vi "Termo_1.5__.vi"() -> ()   [LabVIEW 2013]
doc: "Программа мониторинга температуры"
uses:
  <vilib>/Utility/error.llb/DialogType.ctl
panel:
  out "Связь с прибором":bool
  out "Configuring ADC?":bool
  in  "Tab Control":enum32{"Измерения", "Настройки", "Kоэффициенты"}(tab)
  in  "Autoscale":bool=TRUE
  out "часы":string="0"
  in  "Т max":u16=300 min=2 max=500 step=1
  in  "Т min":u16=3 min=1 max=350
  out "T2":dbl format="%.2f"
  out "T4":dbl format="%.2f"
  out "T1":dbl format="%.2f"
  out "T3":dbl format="%.2f"
  out "T6":dbl format="%.2f"
  out "T8":dbl format="%.2f"
  out "T5":dbl format="%.2f"
  out "T7":dbl format="%.2f"
  out "disconnected":bool
  in  "Добавить время":dbl(ring)=300.0 items=["1 мин."=60.0, "5 мин."=300.0, "20 мин."=1200.0]
  in  "Стоп измер.":bool
  in  "Старт измер.":bool
  in  "stop":bool
  out "R2":dbl format="%.2f"
  out "R4":dbl format="%.2f"
  out "R1":dbl format="%.2f"
  out "R3":dbl format="%.2f"
  out "мин.":string="1"
  in  "xScale +":bool
  in  "xScale -":bool
  in  "R max":u16=6000 min=2 max=10000 step=1
  in  "R min":u16=100 min=1 max=350
  in  "GraphLookB":bool
  out "R6":dbl format="%.2f"
  out "R8":dbl format="%.2f"
  out "R5":dbl format="%.2f"
  out "R7":dbl format="%.2f"
  in  "1_ch_visible":bool=TRUE
  in  "2_ch_visible":bool=TRUE
  in  "3_ch_visible":bool=TRUE
  in  "4_ch_visible":bool=TRUE
  in  "5_ch_visible":bool=TRUE
  in  "6_ch_visible":bool=TRUE
  in  "7_ch_visible":bool=TRUE
  in  "8_ch_visible":bool=TRUE
  in  "ADC_dyn_range":T1(ring)=enum."± 0.625 В"
  out "История операций":string
  in  "Buf_size":u8=16 min=1 max=128
  in  "SPS":T2(ring)
  in  "disconnect":bool
  in  "connect":bool
  in  "IP-адрес":string="192.168.127.254"
  in  "порт":u16=4001
  out "Расположение\n файла":path caption="Расположение файла"
  in  "load_coeff.":bool caption="Disconn"
  in  "save_coeff.":bool caption="Disconn"
  in  "Coeff_cl_ch8":T3 caption="Канал 8" {"R" format="%#_16g"; "k7" format="%#_16g"; "k6" format="%#_16g"; "k5" format="%#_16g"; "k4" format="%#_16g"; "k3" format="%#_16g"; "k2" format="%#_16g"; "k1" format="%#_16g"}
  in  "Coeff_cl_ch7":T3 caption="Канал 7" {"R" format="%#_16g"; "k7" format="%#_16g"; "k6" format="%#_16g"; "k5" format="%#_16g"; "k4" format="%#_16g"; "k3" format="%#_16g"; "k2" format="%#_16g"; "k1" format="%#_16g"}
  in  "Coeff_cl_ch6":T3 caption="Канал 6" {"R" format="%#_16g"; "k7" format="%#_16g"; "k6" format="%#_16g"; "k5" format="%#_16g"; "k4" format="%#_16g"; "k3" format="%#_16g"; "k2" format="%#_16g"; "k1" format="%#_16g"}
  in  "Coeff_cl_ch5":T3 caption="Канал 5" {"R" format="%#_16g"; "k7" format="%#_16g"; "k6" format="%#_16g"; "k5" format="%#_16g"; "k4" format="%#_16g"; "k3" format="%#_16g"; "k2" format="%#_16g"; "k1" format="%#_16g"}
  in  "Coeff_cl_ch4":T3 caption="Канал 4" {"R" format="%#_16g"; "k7" format="%#_16g"; "k6" format="%#_16g"; "k5" format="%#_16g"; "k4" format="%#_16g"; "k3" format="%#_16g"; "k2" format="%#_16g"; "k1" format="%#_16g"}
  in  "Coeff_cl_ch3":T3 caption="Канал 3" {"R" format="%#_16g"; "k7" format="%#_16g"; "k6" format="%#_16g"; "k5" format="%#_16g"; "k4" format="%#_16g"; "k3" format="%#_16g"; "k2" format="%#_16g"; "k1" format="%#_16g"}
  in  "Coeff_cl_ch2":T3 caption="Канал 2" {"R" format="%#_16g"; "k7" format="%#_16g"; "k6" format="%#_16g"; "k5" format="%#_16g"; "k4" format="%#_16g"; "k3" format="%#_16g"; "k2" format="%#_16g"; "k1" format="%#_16g"}
  in  "Coeff_cl_ch1":T3 caption="Канал 1" {"R" format="%#_16g"; "k7" format="%#_16g"; "k6" format="%#_16g"; "k5" format="%#_16g"; "k4" format="%#_16g"; "k3" format="%#_16g"; "k2" format="%#_16g"; "k1" format="%#_16g"}
  out "Сутки":string
  out "счетчик":u32=4001
  in  "Запись в файл":bool
  out "сек.":string="0"
  out "Graphs T":dynamicdata(graph) caption="Температура, К"
  out "refnum out":refnum<file>
  in  "File header exist?":bool caption="Disconn"
  out "connection ID":refnum<k5>
  out "Graphs R":dynamicdata(graph) caption="Сопротивление, Ом"
  out "Расположение файла":path
  # "T [K]"
  # "Канал"
  # "R [Ом]"
  # "1"
  # "2"
  # "3"
  # "4"
  # "5"
  # "6"
  # "7"
  # "8"
  # "Измерения"
  # "Шкала Т"
  # "Шкала R"
  # "Интервал просмотра"
  # ":"
  # "Скорость измерений"
  # "SPS = Samples Per Second"
  # "Динамический диапазон"
  # "Размер буфера усреднения"
  # "Подключение"
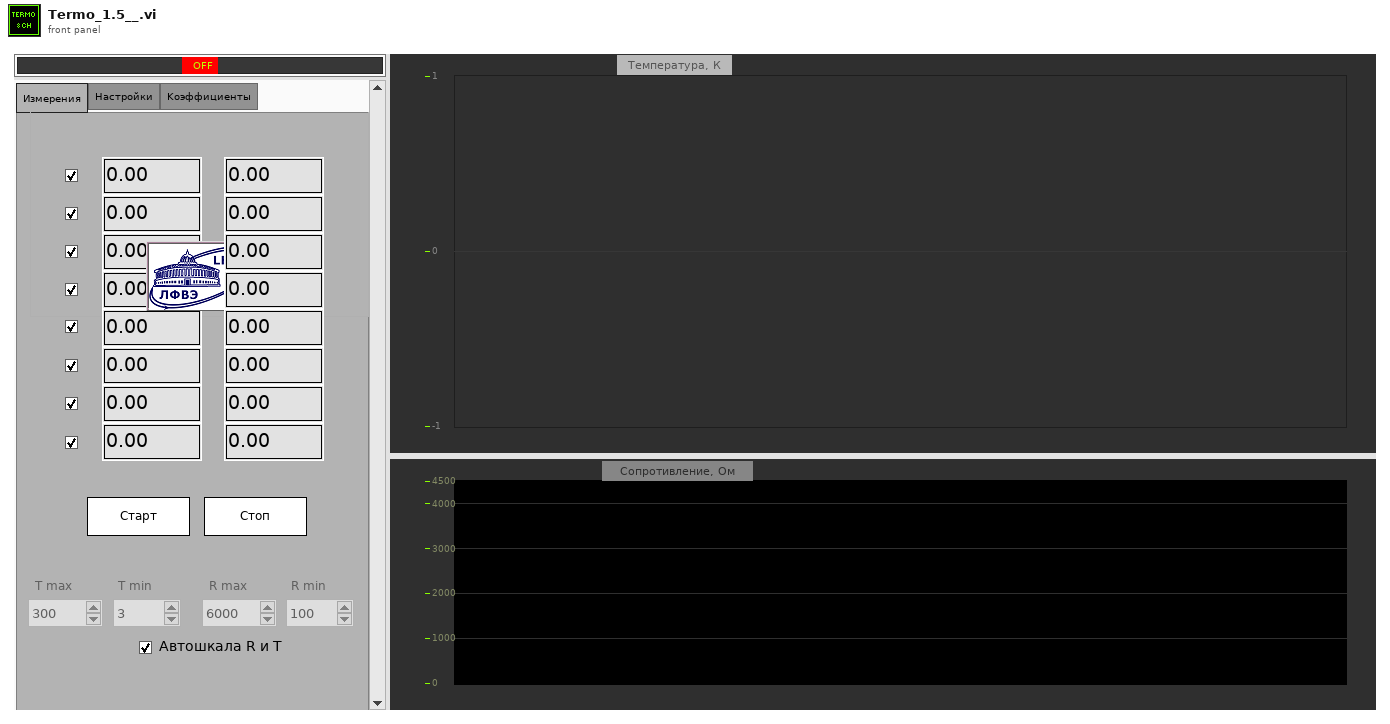
[diagram p1: front panel]
types:
  T1 = enum16{"± 5 В", "± 2.5 В", "± 1.25 В", "± 0.625 В", "± 312.5 мВ", "± 156.25 мВ", "± 78.125 мВ"}
  T2 = enum16{"2,5 SPS", "5 SPS", "10 SPS", "25 SPS", "50 SPS", "100 SPS", "500 SPS", "1 kSPS", "3,75 kSPS"}
  T3 = cluster{"k1":ext, "k2":ext, "k3":ext, "k4":ext, "k5":ext, "k6":ext, "k7":ext, "R":ext}
  T4 = enum32{"Page Enabled", "Page Disabled", "Page Disabled & Grayed"}
  T5 = enum16{"Standard", "Buffered", "CRLF", "Immediate"}
  T6 = typedef "DialogType.ctl" = u16
  T7 = typedef "LVDateTimeRec.ctl" = cluster{"fractional second":dbl, "second":i32, "minute":i32, "hour":i32, "day of month":i32, "month":i32, "year":i32, "day of week":i32, "day of year":i32, "DST":i32}
  T8 = cluster{" R1":dbl, " R2":dbl, " R3":dbl, " R4":dbl, " R5":dbl, "R6":dbl, " R7":dbl, "R8":dbl}
  T9 = cluster{" T1":dbl, "T2":dbl, "T3":dbl, "T4":dbl, " T5":dbl, "T6":dbl, "T7":dbl, "T8":dbl}
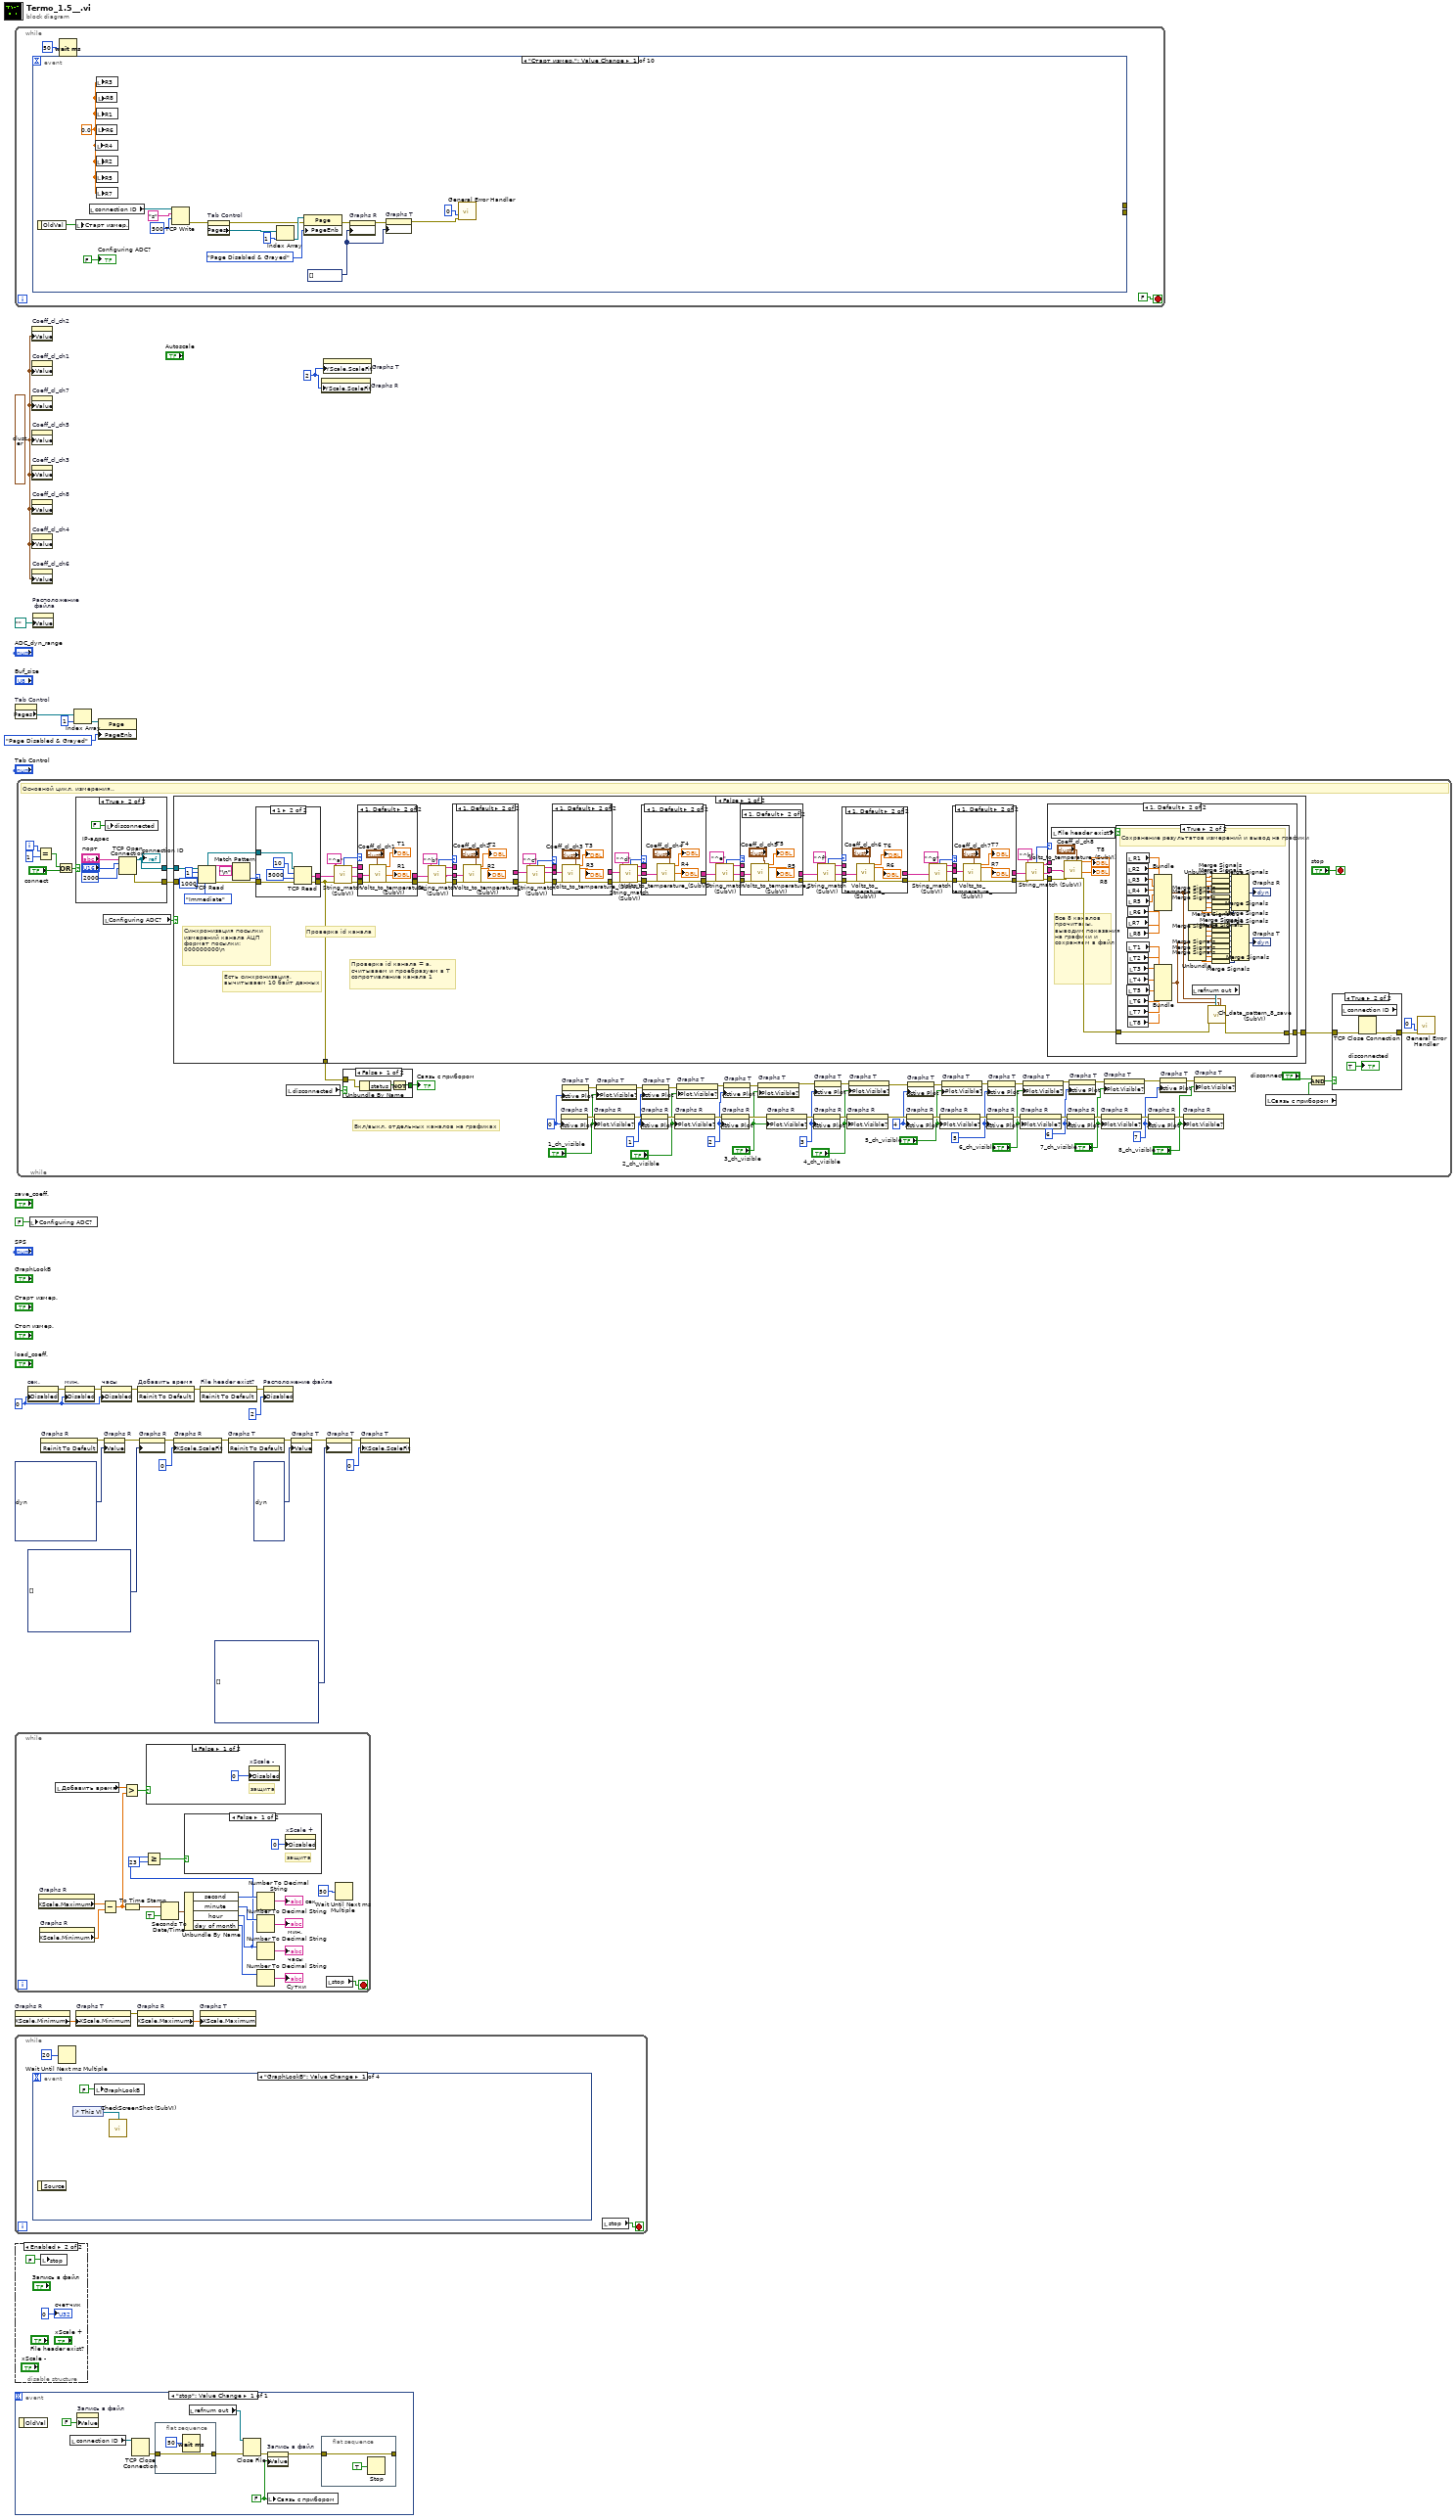
[diagram p0: block diagram]
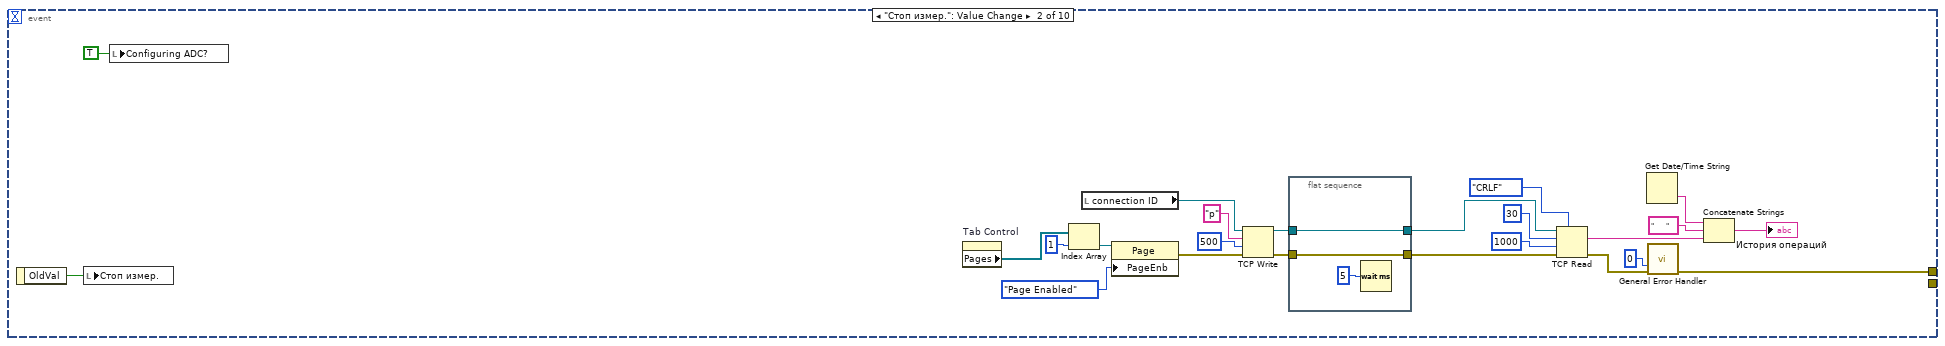
[diagram p2: hidden frame]
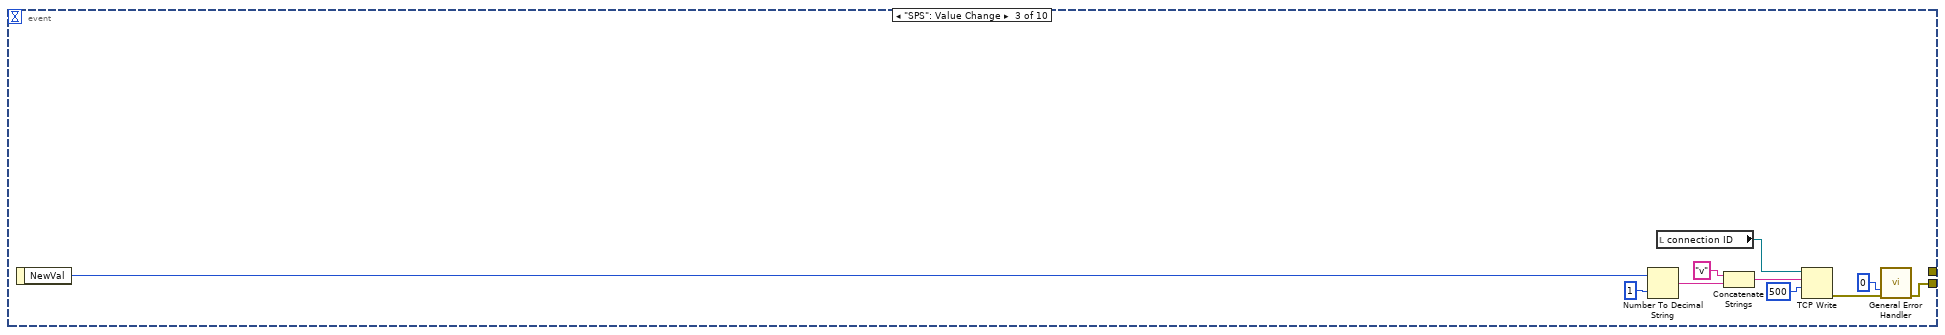
[diagram p3: hidden frame]
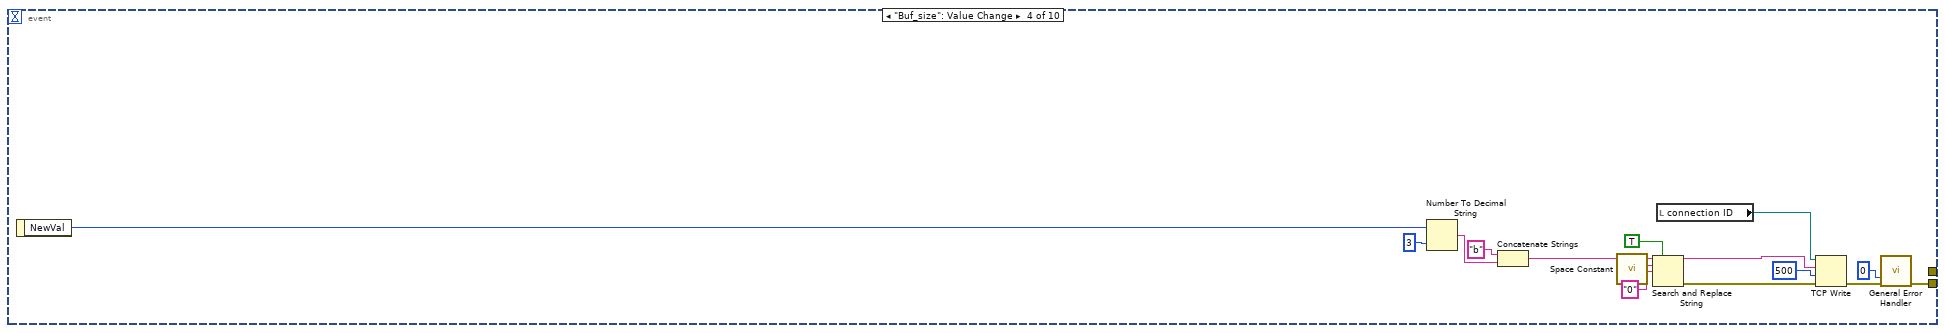
[diagram p4: hidden frame]
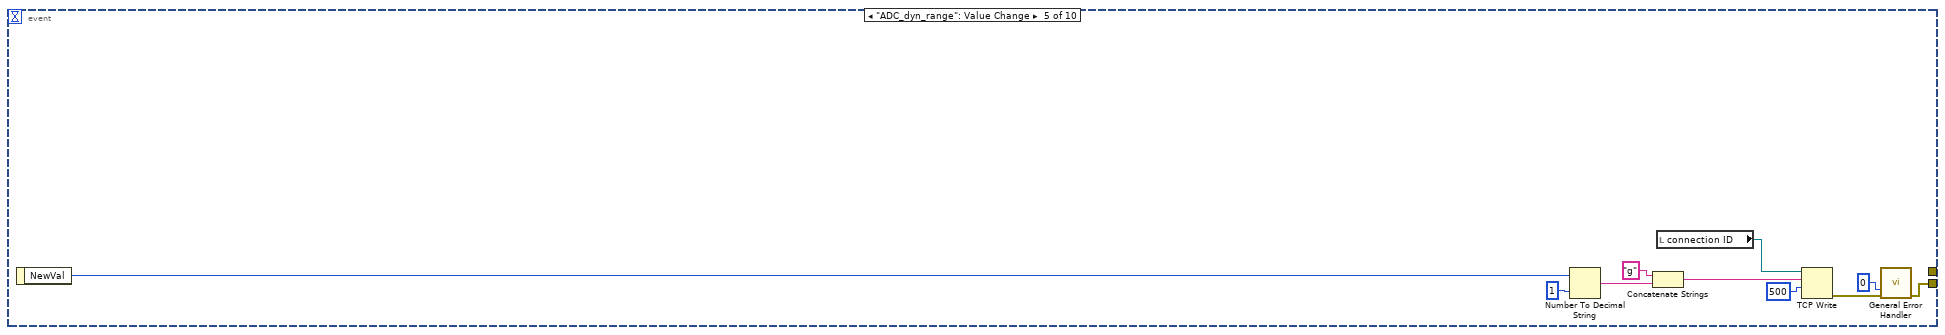
[diagram p5: hidden frame]
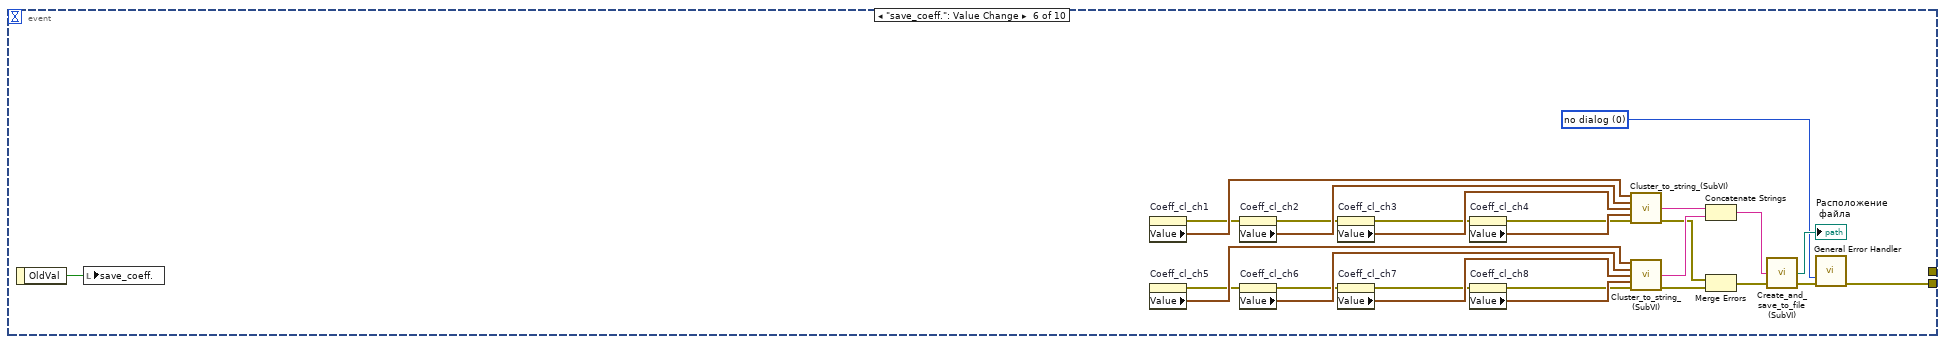
[diagram p6: hidden frame]
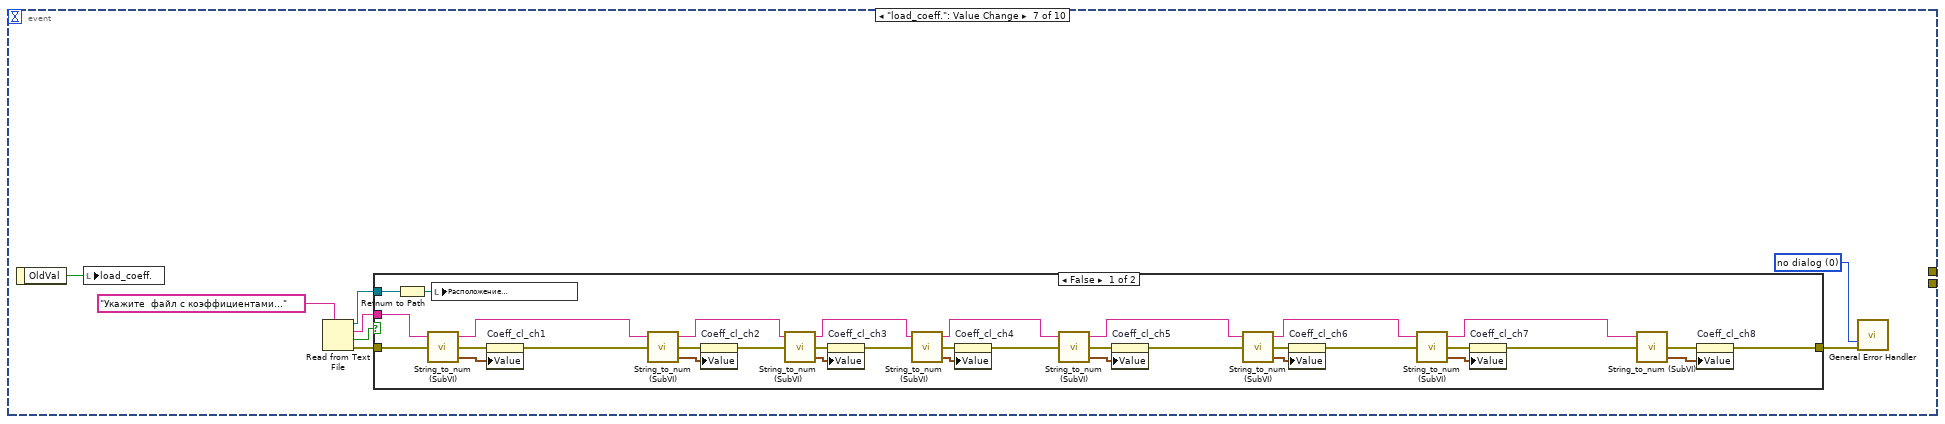
[diagram p7: hidden frame]
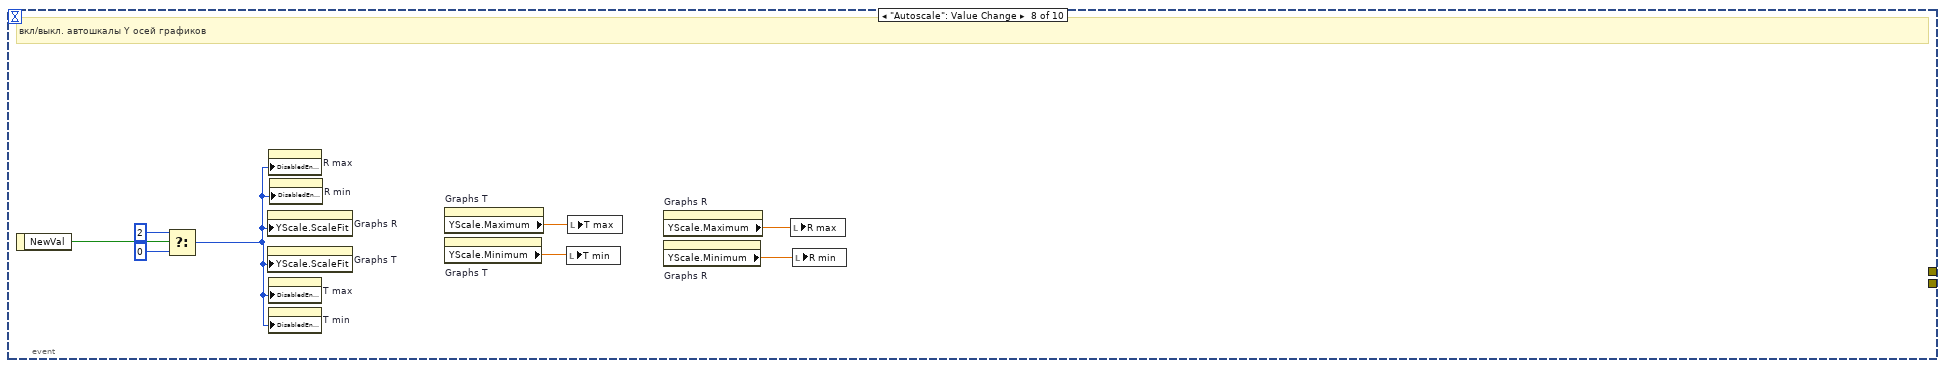
[diagram p9: hidden frame]
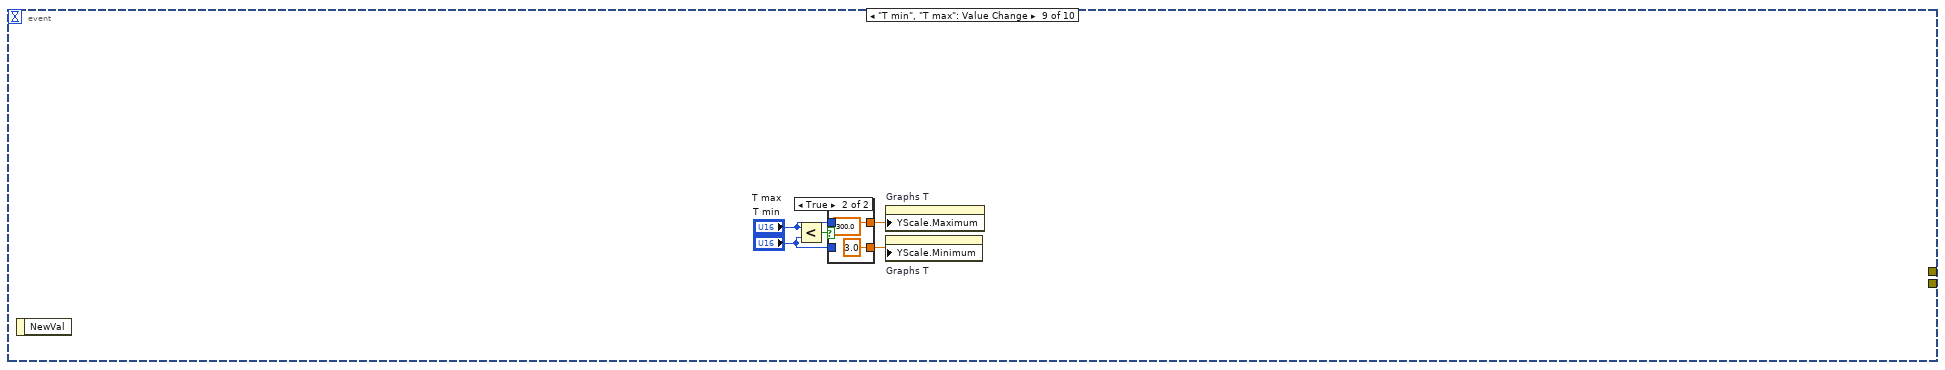
[diagram p10: hidden frame]
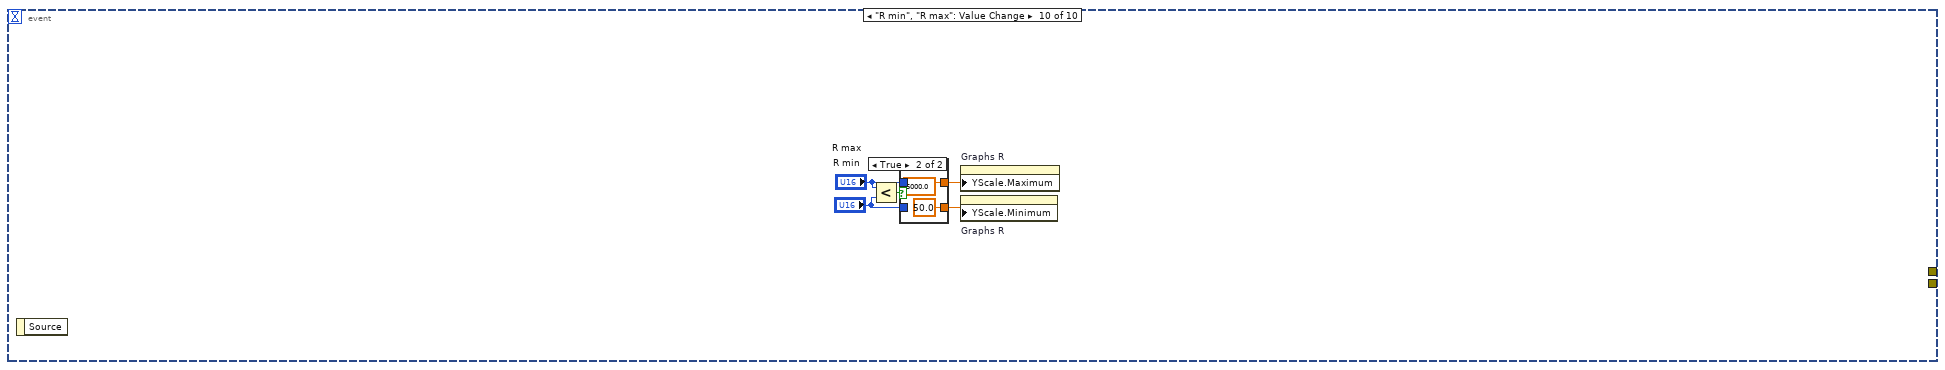
[diagram p12: hidden frame]
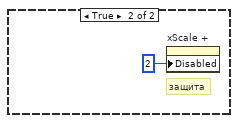
[diagram p14: hidden frame]
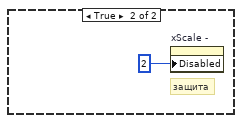
[diagram p15: hidden frame]
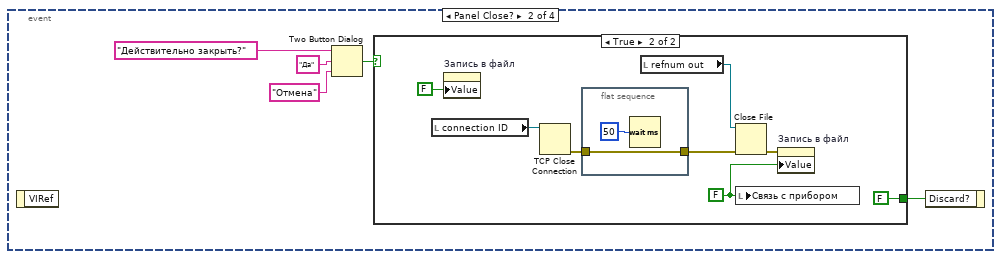
[diagram p17: hidden frame]
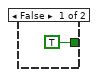
[diagram p18: hidden frame]
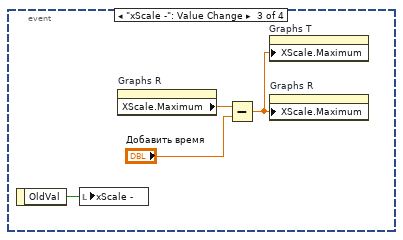
[diagram p19: hidden frame]
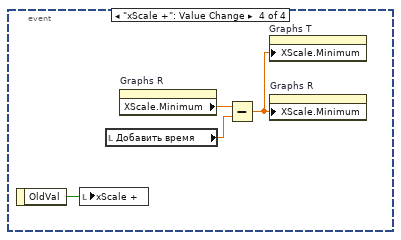
[diagram p20: hidden frame]
diagram:
  w1 = u8 2 ("Y Scale.Scale Fit")
  w3 = T3 {"k1"=0.0, "k2"=0.0, "k3"=0.0, "k4"=0.0, "k5"=0.0, "k6"=0.0, "k7"=0.0, "R"=0.0} ("Coeff_cl_ch2")
  w30 = u8 0 ("Disabled")
  n1 = while {
    stop <- FALSE stop-if-true
    n2 = event shown="[0] \"Старт измер.\": Value Change" {
      selector: _ -> [_ _ _ _ _ _ _ _ _ _]
      dyn-events: _ -> [_ _ _ _ _ _ _ _ _ _]
      timeout: _ -> [_ _ _ _ _ _ _ _ _ _]
      tunnel: [_ w53 _ _ _ _ _ _ _ _] -> _
      tunnel: [_ _ w79 w89 w103 w114 _ _ _ _] -> _
      event "Старт измер.": Value Change {
        w41 = 0.0 ("3")
        w35 = dynamicdata[] [] ("History Data")
        n3 = event-data() -> ("OldVal"=w50:bool)  [unwired: 1 in]
        n4 = local write "Старт измер."(w50) -> ()
        n5 = local read "connection ID"() -> (w46:refnum<k5>)
        n6 = local write "R4"(w41) -> ()
        n7 = local write "R3"(w41) -> ()
        n8 = local write "R1"(w41) -> ()
        n9 = local write "R2"(w41) -> ()
        n10 = local write "R5"(w41) -> ()
        n11 = local write "R7"(w41) -> ()
        n12 = local write "R8"(w41) -> ()
        n13 = local write "R6"(w41) -> ()
        n14 = TCP Write(connection ID=w46, data in="s", 9:500 ("timeout ms (25000)")) -> (error out=w39:errorcluster)  [unwired: 1 in, 2 out]
        n15 = property on="Tab Control" class="TabCtl (strict)"(error in=w39) -> (error out=w38:errorcluster, "Pages"=w45:refnum<vi>[])  [unwired: 1 in, 1 out]
        n16 = Index Array(array=w45, index=1) -> (element=w44:refnum<vi>)
        n17 = property class="Page"(reference=w44, error in=w38, "PageEnb"=T4."Page Disabled & Grayed" ("Page Enabled State")) -> (error out=w40:errorcluster)  [unwired: 1 out]
        n18 = property on="Graphs R" class="WFChart (strict)"(error in=w40, "History Data"=w35) -> (error out=w36:errorcluster)  [unwired: 1 in, 1 out]
        n19 = property on="Graphs T" class="WFChart (strict)"(error in=w36, "History Data"=w35) -> (error out=w34:errorcluster)  [unwired: 1 in, 1 out]
        n20 = call <vilib>:"General Error Handler.vi"("type of dialog (OK msg:1)"=0 ("timeout ms (25000)"), "error in (no error)"=w34) -> ()  [unwired: 9 in, 5 out]
        "Configuring ADC?" <- FALSE ("TCP_Wr_fl")
      }
      event "Стоп измер.": Value Change {
        n21 = event-data() -> ("OldVal"=w74:bool)  [unwired: 1 in]
        n22 = local write "Стоп измер."(w74) -> ()
        n23 = local write "Configuring ADC?"(TRUE ("TCP_Wr_fl")) -> ()
        n24 = property on="Tab Control" class="TabCtl (strict)"() -> ("Pages"=w69:refnum<vi>[])  [unwired: 2 in, 2 out]
        n25 = Index Array(array=w69, index=1) -> (element=w68:refnum<vi>)
        n26 = local read "connection ID"() -> (w71:refnum<k5>)
        n27 = property class="Page"(reference=w68, "PageEnb"=T4."Page Enabled" ("Page Enabled State")) -> (error out=w51:errorcluster)  [unwired: 1 in, 1 out]
        n28 = TCP Write(connection ID=w71, data in="p", error in (no error)=w51, 9:500 ("timeout ms (25000)")) -> (connection ID out=w61:refnum<k5>, error out=w59:errorcluster)  [unwired: 1 out]
        n29 = flat-sequence {
          tunnel: [w76] -> w62
          tunnel: w61 -> [w76]
          tunnel: [w75] -> w60
          tunnel: w59 -> [w75]
          frame #0 {
            n30 = Wait (ms)(milliseconds to wait=u32 5) -> ()  [unwired: 1 out]
          }
        }
        n31 = TCP Read(connection ID=w62, bytes to read=30, error in (no error)=w60, 7:T5."CRLF" ("mode (standard)"), 9:1000 ("timeout ms (25000)")) -> (data out=w56:string, error out=w54:errorcluster)  [unwired: 1 out]
        n32 = Get Date/Time String() -> (time string=w58:string)  [unwired: 3 in, 1 out]
        n33 = call <vilib>:"General Error Handler.vi"("type of dialog (OK msg:1)"=0 ("timeout ms (25000)"), "error in (no error)"=w54) -> ("error out"=w53:errorcluster)  [unwired: 9 in, 4 out]
        n34 = Concatenate Strings(w58, "      " ("string"), w56) -> (→"История операций":string)
      }
      event "SPS": Value Change {
        n35 = event-data() -> ("NewVal"=w84:T2)  [unwired: 1 in]
        n36 = Number To Decimal String(number=w84, width (-)=i16 1) -> (decimal integer string=w82:string)
        n37 = local read "connection ID"() -> (w86:refnum<k5>)
        n38 = Concatenate Strings("v" ("data in"), w82) -> (w81:string)
        n39 = TCP Write(connection ID=w86, data in=w81, 9:500 ("timeout ms (25000)")) -> (error out=w80:errorcluster)  [unwired: 1 in, 2 out]
        n40 = call <vilib>:"General Error Handler.vi"("type of dialog (OK msg:1)"=0 ("timeout ms (25000)"), "error in (no error)"=w80) -> ("error out"=w79:errorcluster)  [unwired: 9 in, 4 out]
      }
      event "Buf_size": Value Change {
        n41 = event-data() -> ("NewVal"=w99:u8)  [unwired: 1 in]
        n42 = Number To Decimal String(number=w99, width (-)=i16 3) -> (decimal integer string=w97:string)
        n43 = Concatenate Strings("b" ("data in"), w97) -> (w96:string)
        n44 = call <vilib>:"Space Constant.vi"() -> ("String"=w94:string)
        n45 = Search and Replace String(replace all?=TRUE ("replace all? (F)"), input string=w96, search string=w94, replace string="0" ("replace string (\"\")")) -> (result string=w95:string, error out=w91:errorcluster)  [unwired: 4 in, 2 out]
        n46 = local read "connection ID"() -> (w101:refnum<k5>)
        n47 = TCP Write(connection ID=w101, data in=w95, error in (no error)=w91, 9:500 ("timeout ms (25000)")) -> (error out=w90:errorcluster)  [unwired: 2 out]
        n48 = call <vilib>:"General Error Handler.vi"("type of dialog (OK msg:1)"=0 ("timeout ms (25000)"), "error in (no error)"=w90) -> ("error out"=w89:errorcluster)  [unwired: 9 in, 4 out]
      }
      event "ADC_dyn_range": Value Change {
        n49 = event-data() -> ("NewVal"=w109:T1)  [unwired: 1 in]
        n50 = Number To Decimal String(number=w109, width (-)=i16 1) -> (decimal integer string=w107:string)
        n51 = Concatenate Strings("g" ("data in"), w107) -> (w106:string)
        n52 = local read "connection ID"() -> (w111:refnum<k5>)
        n53 = TCP Write(connection ID=w111, data in=w106, 9:500 ("timeout ms (25000)")) -> (error out=w104:errorcluster)  [unwired: 1 in, 2 out]
        n54 = call <vilib>:"General Error Handler.vi"("type of dialog (OK msg:1)"=0 ("timeout ms (25000)"), "error in (no error)"=w104) -> ("error out"=w103:errorcluster)  [unwired: 9 in, 4 out]
      }
      event "save_coeff.": Value Change {
        w113 = T6 0 items=["no dialog", "OK message", "continue or stop message", "OK message + warnings", "continue/stop + warnings"] ("type of dialog (OK msg:1)")
        n55 = event-data() -> ("OldVal"=w120:bool)  [unwired: 1 in]
        n56 = local write "save_coeff."(w120) -> ()
        n57 = property on="Coeff_cl_ch1" class="Clust (strict)"() -> (error out=w127:errorcluster, "Value"=w135:T3)  [unwired: 2 in, 1 out]
        n58 = property on="Coeff_cl_ch5" class="Clust (strict)"() -> (error out=w124:errorcluster, "Value"=w131:T3)  [unwired: 2 in, 1 out]
        n59 = property on="Coeff_cl_ch2" class="Clust (strict)"(error in=w127) -> (error out=w126:errorcluster, "Value"=w134:T3)  [unwired: 1 in, 1 out]
        n60 = property on="Coeff_cl_ch6" class="Clust (strict)"(error in=w124) -> (error out=w123:errorcluster, "Value"=w130:T3)  [unwired: 1 in, 1 out]
        n61 = property on="Coeff_cl_ch3" class="Clust (strict)"(error in=w126) -> (error out=w125:errorcluster, "Value"=w133:T3)  [unwired: 1 in, 1 out]
        n62 = property on="Coeff_cl_ch7" class="Clust (strict)"(error in=w123) -> (error out=w122:errorcluster, "Value"=w129:T3)  [unwired: 1 in, 1 out]
        n63 = property on="Coeff_cl_ch4" class="Clust (strict)"(error in=w125) -> (error out=w117:errorcluster, "Value"=w132:T3)  [unwired: 1 in, 1 out]
        n64 = property on="Coeff_cl_ch8" class="Clust (strict)"(error in=w122) -> (error out=w116:errorcluster, "Value"=w128:T3)  [unwired: 1 in, 1 out]
        n65 = call "Cluster_to_string_(SubVI).vi"("input cluster 1"=w135, "input cluster 2"=w134, "input cluster 3"=w133, "input cluster 4"=w132, "error in"=w117) -> ("string of coefficients"=w138:string, "error out"=w119:errorcluster)  [unwired: 9 in]
        n66 = call "Cluster_to_string_(SubVI).vi"("input cluster 1"=w131, "input cluster 2"=w130, "input cluster 3"=w129, "input cluster 4"=w128, "error in"=w116) -> ("string of coefficients"=w139:string, "error out"=w118:errorcluster)  [unwired: 9 in]
        n67 = Concatenate Strings(w138, w139) -> (w121:string)
        n68 = Merge Errors(w119, w118) -> (w137:errorcluster)
        n69 = call "Create_and_save_to_file (SubVI).vi"("input string"=w121, "error in"=w137) -> ("Текущее расположение файла"=→"Расположение\n файла":path, "error out"=w115:errorcluster)  [unwired: 4 in]
        n70 = call <vilib>:"General Error Handler.vi"("type of dialog (OK msg:1)"=w113, "error in (no error)"=w115) -> ("error out"=w114:errorcluster)  [unwired: 9 in, 4 out]
      }
      event "load_coeff.": Value Change {
        w141 = T6 0 items=["no dialog", "OK message", "continue or stop message", "OK message + warnings", "continue/stop + warnings"] ("type of dialog (OK msg:1)")
        n71 = event-data() -> ("OldVal"=w147:bool)  [unwired: 1 in]
        n72 = local write "load_coeff."(w147) -> ()
        n73 = Read from Text File(prompt (Open existing file)="Укажите  файл с коэффициентами...") -> (refnum out=w140:refnum<file>, text=w144:string, cancelled=w143:bool, error out=w145:errorcluster)  [unwired: 3 in]
        n74 = case shown="False" w143 {
          tunnel: w145 -> [w182 w183]
          tunnel: w144 -> [w181 _]
          tunnel: [w150 w183] -> w142
          tunnel: w140 -> [w149 _]
          frame False {
            n75 = Refnum to Path(1:w149) -> (0:w148:path)
            n76 = call "String_to_num (SubVI).vi"("String in"=w181, "error in"=w182) -> ("Rest of string OUT"=w177:string, "error out"=w179:errorcluster, "output cluster \nof coefficients"=w180:T3)  [unwired: 5 in]
            n77 = local write "Расположение\n файла"(w148) -> ()
            n78 = property on="Coeff_cl_ch1" class="Clust (strict)"(error in=w179, "Value"=w180) -> (error out=w178:errorcluster)  [unwired: 1 in, 1 out]
            n79 = call "String_to_num (SubVI).vi"("String in"=w177, "error in"=w178) -> ("Rest of string OUT"=w173:string, "error out"=w176:errorcluster, "output cluster \nof coefficients"=w175:T3)  [unwired: 5 in]
            n80 = property on="Coeff_cl_ch2" class="Clust (strict)"(error in=w176, "Value"=w175) -> (error out=w174:errorcluster)  [unwired: 1 in, 1 out]
            n81 = call "String_to_num (SubVI).vi"("String in"=w173, "error in"=w174) -> ("Rest of string OUT"=w170:string, "error out"=w172:errorcluster, "output cluster \nof coefficients"=w171:T3)  [unwired: 5 in]
            n82 = property on="Coeff_cl_ch3" class="Clust (strict)"(error in=w172, "Value"=w171) -> (error out=w169:errorcluster)  [unwired: 1 in, 1 out]
            n83 = call "String_to_num (SubVI).vi"("String in"=w170, "error in"=w169) -> ("Rest of string OUT"=w165:string, "error out"=w168:errorcluster, "output cluster \nof coefficients"=w167:T3)  [unwired: 5 in]
            n84 = property on="Coeff_cl_ch4" class="Clust (strict)"(error in=w168, "Value"=w167) -> (error out=w166:errorcluster)  [unwired: 1 in, 1 out]
            n85 = call "String_to_num (SubVI).vi"("String in"=w165, "error in"=w166) -> ("Rest of string OUT"=w161:string, "error out"=w163:errorcluster, "output cluster \nof coefficients"=w164:T3)  [unwired: 5 in]
            n86 = property on="Coeff_cl_ch5" class="Clust (strict)"(error in=w163, "Value"=w164) -> (error out=w162:errorcluster)  [unwired: 1 in, 1 out]
            n87 = call "String_to_num (SubVI).vi"("String in"=w161, "error in"=w162) -> ("Rest of string OUT"=w157:string, "error out"=w159:errorcluster, "output cluster \nof coefficients"=w160:T3)  [unwired: 5 in]
            n88 = property on="Coeff_cl_ch6" class="Clust (strict)"(error in=w159, "Value"=w160) -> (error out=w158:errorcluster)  [unwired: 1 in, 1 out]
            n89 = call "String_to_num (SubVI).vi"("String in"=w157, "error in"=w158) -> ("Rest of string OUT"=w154:string, "error out"=w155:errorcluster, "output cluster \nof coefficients"=w156:T3)  [unwired: 5 in]
            n90 = property on="Coeff_cl_ch7" class="Clust (strict)"(error in=w155, "Value"=w156) -> (error out=w153:errorcluster)  [unwired: 1 in, 1 out]
            n91 = call "String_to_num (SubVI).vi"("String in"=w154, "error in"=w153) -> ("error out"=w151:errorcluster, "output cluster \nof coefficients"=w152:T3)  [unwired: 5 in, 1 out]
            n92 = property on="Coeff_cl_ch8" class="Clust (strict)"(error in=w151, "Value"=w152) -> (error out=w150:errorcluster)  [unwired: 1 in, 1 out]
          }
          frame True {
          }
        }
        n93 = call <vilib>:"General Error Handler.vi"("type of dialog (OK msg:1)"=w141, "error in (no error)"=w142) -> ()  [unwired: 9 in, 5 out]
      }
      event "Autoscale": Value Change {
        # "вкл/выкл. автошкалы Y осей графиков"
        n94 = event-data() -> ("NewVal"=w191:bool)  [unwired: 1 in]
        n95 = Select(t=u8 2 ("Y Scale.Scale Fit"), s=w191, f=u8 0 ("Y Scale.Scale Fit")) -> (s? t:f=w188:u8)
        n96 = property on="Graphs R" class="WFChart (strict)"("YScale.ScaleFit"=w188) -> ()  [unwired: 2 in, 2 out]
        n97 = property on="Graphs T" class="WFChart (strict)"("YScale.ScaleFit"=w188) -> ()  [unwired: 2 in, 2 out]
        n98 = property on="R max" class="DigNum (strict)"("DisabledEnum"=w188) -> ()  [unwired: 2 in, 2 out]
        n99 = property on="Т max" class="DigNum (strict)"("DisabledEnum"=w188) -> ()  [unwired: 2 in, 2 out]
        n100 = property on="Т min" class="DigNum (strict)"("DisabledEnum"=w188) -> ()  [unwired: 2 in, 2 out]
        n101 = property on="R min" class="DigNum (strict)"("DisabledEnum"=w188) -> ()  [unwired: 2 in, 2 out]
        n102 = property on="Graphs T" class="WFChart (strict)"() -> ("YScale.Maximum"=w184:dbl)  [unwired: 2 in, 2 out]
        n103 = property on="Graphs T" class="WFChart (strict)"() -> ("YScale.Minimum"=w185:dbl)  [unwired: 2 in, 2 out]
        n104 = local write "Т min"(w185) -> ()
        n105 = local write "Т max"(w184) -> ()
        n106 = property on="Graphs R" class="WFChart (strict)"() -> ("YScale.Maximum"=w186:dbl)  [unwired: 2 in, 2 out]
        n107 = property on="Graphs R" class="WFChart (strict)"() -> ("YScale.Minimum"=w187:dbl)  [unwired: 2 in, 2 out]
        n108 = local write "R max"(w186) -> ()
        n109 = local write "R min"(w187) -> ()
      }
      event "Т min", "Т max": Value Change {
        n110 = event-data() -> ()  [unwired: 1 in, 1 out]
        n111 = Less?(x="Т max", y="Т min") -> (x < y?=w196:bool)
        n112 = case shown="True" w196 {
          tunnel: [w197 300.0 ("x+1")] -> w194
          tunnel: [w198 3.0 ("x+1")] -> w195
          tunnel: "Т max" -> [w197 _]
          tunnel: "Т min" -> [w198 _]
          frame False {
          }
          frame True {
          }
        }
        n113 = property on="Graphs T" class="WFChart (strict)"("YScale.Maximum"=w194) -> ()  [unwired: 2 in, 2 out]
        n114 = property on="Graphs T" class="WFChart (strict)"("YScale.Minimum"=w195) -> ()  [unwired: 2 in, 2 out]
      }
      event "R min", "R max": Value Change {
        n115 = event-data() -> ()  [unwired: 1 in, 1 out]
        n116 = Less?(x="R max", y="R min") -> (x < y?=w203:bool)
        n117 = case shown="True" w203 {
          tunnel: [w206 5000.0 ("x+1")] -> w205
          tunnel: [w207 50.0 ("x+1")] -> w204
          tunnel: "R max" -> [w206 _]
          tunnel: "R min" -> [w207 _]
          frame False {
          }
          frame True {
          }
        }
        n118 = property on="Graphs R" class="WFChart (strict)"("YScale.Maximum"=w205) -> ()  [unwired: 2 in, 2 out]
        n119 = property on="Graphs R" class="WFChart (strict)"("YScale.Minimum"=w204) -> ()  [unwired: 2 in, 2 out]
      }
    }
    n120 = Wait (ms)(milliseconds to wait=u32 50) -> ()  [unwired: 1 out]
  }
  n121 = property on="Tab Control" class="TabCtl (strict)"() -> ("Pages"=w15:refnum<vi>[])  [unwired: 2 in, 2 out]
  n122 = while {
    stop <- w229 stop-if-true
    n123 = property on="Graphs R" class="WFChart (strict)"() -> ("XScale.Maximum"=w228:dbl)  [unwired: 2 in, 2 out]
    n124 = property on="Graphs R" class="WFChart (strict)"() -> ("XScale.Minimum"=w227:dbl)  [unwired: 2 in, 2 out]
    n125 = local read "Добавить время"() -> (w225:dbl)
    n126 = Subtract(x=w228, y=w227) -> (x-y=w214:dbl)
    n127 = Greater?(x=w225, y=w214) -> (0:w226:bool)
    n128 = To Time Stamp(1:w214) -> (0:w223:timestamp)
    n129 = case shown="False" w226 {
      frame False {
        # "защита"
        n130 = property on="xScale -" class="Bool (strict)"("Disabled"=u8 0) -> ()  [unwired: 2 in, 2 out]
      }
      frame True {
        # "защита"
        n131 = property on="xScale -" class="Bool (strict)"("Disabled"=u8 2) -> ()  [unwired: 2 in, 2 out]
      }
    }
    n132 = Seconds To Date/Time(time stamp (now)=w223, to UTC (F)=TRUE) -> (date time rec=w222:T7)
    n133 = Unbundle By Name(w222) -> ("second"=w221:i32, "minute"=w220:i32, "hour"=w211:i32, "day of month"=w219:i32)
    n134 = Greater Or Equal?(x=w211, y=23) -> (x >= y?=w212:bool)
    n135 = case shown="False" w212 {
      frame False {
        # "защита"
        n136 = property on="xScale +" class="Bool (strict)"("Disabled"=u8 0) -> ()  [unwired: 2 in, 2 out]
      }
      frame True {
        # "защита"
        n137 = property on="xScale +" class="Bool (strict)"("Disabled"=u8 2) -> ()  [unwired: 2 in, 2 out]
      }
    }
    n138 = Number To Decimal String(number=w221) -> (decimal integer string=→"сек.":string)  [unwired: 1 out]
    n139 = Number To Decimal String(number=w220) -> (decimal integer string=→"мин.":string)  [unwired: 1 out]
    n140 = Number To Decimal String(number=w211) -> (decimal integer string=→"часы":string)  [unwired: 1 out]
    n141 = Number To Decimal String(number=w219) -> (decimal integer string=→"Сутки":string)  [unwired: 1 out]
    n142 = local read "stop"() -> (w229:bool)
    n143 = Wait Until Next ms Multiple(millisecond multiple=u32 50) -> ()  [unwired: 1 out]
  }
  n144 = property on="Graphs R" class="WFChart (strict)"() -> ("XScale.Minimum"=w6:dbl)  [unwired: 2 in, 2 out]
  n145 = while {
    stop <- w234 stop-if-true
    n146 = event shown="[0] \"GraphLookB\": Value Change" {
      selector: _ -> [_ _ _ _]
      dyn-events: _ -> [_ _ _ _]
      timeout: _ -> [_ _ _ _]
      event "GraphLookB": Value Change {
        n147 = event-data() -> ()  [unwired: 2 out]
        n148 = control-ref of="This VI"() -> (w236:refnum<vi>)
        n149 = local write "GraphLookB"(FALSE ("Снимок")) -> ()
        n150 = call "CheckScreenShot (SubVI).vi"("VI reference"=w236) -> ()  [unwired: 15 in]
      }
      event Panel Close? {
        n151 = event-data() -> ()  [unwired: 2 out]
        n152 = Two Button Dialog(message="Действительно закрыть?", 1:"Отмена" ("T button name (\"OK\")"), 2:"Да" ("T button name (\"OK\")")) -> (T button?=w242:bool)
        n153 = case shown="True" w242 {
          tunnel: [TRUE ("Discard?") FALSE ("Discard?")] -> w238
          frame False {
          }
          frame True {
            w248 = FALSE ("Запись в файл")
            n154 = local read "connection ID"() -> (w245:refnum<k5>)
            n155 = property on="Запись в файл" class="Bool (strict)"("Value"=FALSE ("Запись в файл")) -> ()  [unwired: 2 in, 2 out]
            n156 = TCP Close Connection(connection ID=w245) -> (error out=w251:errorcluster)  [unwired: 1 in, 2 out]
            n157 = flat-sequence {
              tunnel: [w252] -> w250
              tunnel: w251 -> [w252]
              frame #0 {
                n158 = Wait (ms)(milliseconds to wait=u32 50) -> ()  [unwired: 1 out]
              }
            }
            n159 = local read "refnum out"() -> (w247:refnum<file>)
            n160 = Close File(refnum=w247, error in=w250) -> (error out=w246:errorcluster)  [unwired: 1 out]
            n161 = local write "Связь с прибором"(w248) -> ()
            n162 = property on="Запись в файл" class="Bool (strict)"(error in=w246, "Value"=w248) -> ()  [unwired: 1 in, 2 out]
          }
        }
        n163 = event-data("Discard?"=w238) -> ()  [unwired: 1 in, 1 out]
      }
      event "xScale -": Value Change {
        n164 = event-data() -> ("OldVal"=w256:bool)  [unwired: 1 out]
        n165 = local write "xScale -"(w256) -> ()
        n166 = property on="Graphs R" class="WFChart (strict)"() -> ("XScale.Maximum"=w257:dbl)  [unwired: 2 in, 2 out]
        n167 = Subtract(x=w257, y="Добавить время") -> (x-y=w254:dbl)
        n168 = property on="Graphs T" class="WFChart (strict)"("XScale.Maximum"=w254) -> ()  [unwired: 2 in, 2 out]
        n169 = property on="Graphs R" class="WFChart (strict)"("XScale.Maximum"=w254) -> ()  [unwired: 2 in, 2 out]
      }
      event "xScale +": Value Change {
        n170 = event-data() -> ("OldVal"=w260:bool)  [unwired: 1 out]
        n171 = local write "xScale +"(w260) -> ()
        n172 = local read "Добавить время"() -> (w259:dbl)
        n173 = property on="Graphs R" class="WFChart (strict)"() -> ("XScale.Minimum"=w261:dbl)  [unwired: 2 in, 2 out]
        n174 = Subtract(x=w261, y=w259) -> (x-y=w258:dbl)
        n175 = property on="Graphs T" class="WFChart (strict)"("XScale.Minimum"=w258) -> ()  [unwired: 2 in, 2 out]
        n176 = property on="Graphs R" class="WFChart (strict)"("XScale.Minimum"=w258) -> ()  [unwired: 2 in, 2 out]
      }
    }
    n177 = Wait Until Next ms Multiple(millisecond multiple=u32 20) -> ()  [unwired: 1 out]
    n178 = local read "stop"() -> (w234:bool)
  }
  n179 = disable-structure shown="Enabled" {
    frame Disabled {
    }
    frame Enabled {
      n180 = local write "stop"(FALSE ("Boolean")) -> ()
      "счетчик" <- u32 0 ("счетчик")
    }
  }
  n181 = event shown="[0] \"stop\": Value Change" {
    selector: _ -> [_]
    dyn-events: _ -> [_]
    timeout: _ -> [_]
    event "stop": Value Change {
      w268 = FALSE ("Запись в файл")
      n182 = event-data() -> ()  [unwired: 1 in, 1 out]
      n183 = local read "connection ID"() -> (w265:refnum<k5>)
      n184 = property on="Запись в файл" class="Bool (strict)"("Value"=FALSE ("Запись в файл")) -> ()  [unwired: 2 in, 2 out]
      n185 = TCP Close Connection(connection ID=w265) -> (error out=w271:errorcluster)  [unwired: 1 in, 2 out]
      n186 = flat-sequence {
        tunnel: [w274] -> w270
        tunnel: w271 -> [w274]
        frame #0 {
          n187 = Wait (ms)(milliseconds to wait=u32 50) -> ()  [unwired: 1 out]
        }
      }
      n188 = local read "refnum out"() -> (w267:refnum<file>)
      n189 = Close File(refnum=w267, error in=w270) -> (error out=w266:errorcluster)  [unwired: 1 out]
      n190 = property on="Запись в файл" class="Bool (strict)"(error in=w266, "Value"=w268) -> (error out=w264:errorcluster)  [unwired: 1 in, 1 out]
      n191 = local write "Связь с прибором"(w268) -> ()
      n192 = flat-sequence {
        tunnel: w264 -> [w273]
        tunnel: [w273] -> _
        frame #0 {
          n193 = Stop(stop? (T)=TRUE) -> ()
        }
      }
    }
  }
  n194 = while {
    i -> [w336]
    stop <- "stop" stop-if-true
    w279 = u32 7 ("Active Plot")
    w281 = u32 6 ("Active Plot")
    w283 = u32 5 ("Active Plot")
    w286 = u32 4 ("Active Plot")
    w296 = u32 3 ("Active Plot")
    w299 = u32 2 ("Active Plot")
    w302 = u32 1 ("Active Plot")
    w307 = u32 0 ("Active Plot")
    # "Вкл/выкл. отдельных каналов на графиках"
    # "Основной цикл, измерения.."
    n195 = Equal?(x=w336, y=1) -> (x = y?=w337:bool)
    n196 = Or(x=w337, y="connect") -> (x .or. y?=w319:bool)
    n197 = case shown="True" w319 {
      tunnel: [_ w351] -> w317
      tunnel: [w349 w352] -> w320
      frame False {
        n198 = local read "connection ID"() -> (w349:refnum<k5>)
      }
      frame True {
        n199 = local write "disconnected"(FALSE ("disconnected")) -> ()
        n200 = TCP Open Connection(address="IP-адрес", remote port or service name="порт", timeout ms (60000)=2000) -> (connection ID=w352:refnum<k5>, error out=w351:errorcluster)  [unwired: 1 in, 1 out]
        "connection ID" <- w352
      }
    }
    n201 = local read "Configuring ADC?"() -> (w311:bool)
    n202 = case shown="False" w311 {
      tunnel: [w356 w555] -> w277
      tunnel: w317 -> [w417 w555]
      tunnel: w320 -> [w416 _]
      tunnel: [w357 w555] -> w309
      frame False {
        # "Проверка id канала = a,\nсчитываем и проебразуем в Т\nсопротивление канала 1"
        # "Есть синхронизация, \nвычитываем 10 байт данных"
        # "Проверка id канала"
        # "Синхронизация посылки \nизмерений канала АЦП\nформат посылки:\n000000000\\n"
        n203 = TCP Read(connection ID=w416, bytes to read=1, error in (no error)=w417, 7:T5."Immediate" ("mode (standard)"), 9:1000 ("timeout ms (25000)")) -> (connection ID out=w418:refnum<k5>, data out=w419:string, error out=w409:errorcluster)
        n204 = Match Pattern(string=w419, regular expression="\n") -> (offset past match=w415:i32)  [unwired: 4 out]
        n205 = case shown="1" w415 {
          tunnel: [w548 w554] -> w357
          tunnel: [_ w549] -> w410
          tunnel: w418 -> [_ w553]
          tunnel: w409 -> [w548 w552]
          frame -1, Default {
          }
          frame 1 {
            n206 = TCP Read(connection ID=w553, bytes to read=10, error in (no error)=w552, 9:5000 ("timeout ms (25000)")) -> (data out=w549:string, error out=w554:errorcluster)  [unwired: 2 out]
          }
        }
        n207 = call "String_match (SubVI).vi"("channel id"="^a" ("regular expression"), "input string"=w410, "error in"=w357) -> ("match ?"=w407:i32, "output string"=w404:string, "match substring"=w405:string, "error out"=w406:errorcluster)  [unwired: 13 in]
        n208 = case shown="1, Default" w407 {
          tunnel: [w541 w547] -> w388
          tunnel: w406 -> [w541 w546]
          tunnel: w405 -> [_ w544]
          tunnel: [w540 _] -> w422
          tunnel: w404 -> [w540 _]
          frame -1 {
          }
          frame 1, Default {
            n209 = call "Volts_to_temperature_(SubVI).vi"("ch_data_string"=w544, "error in"=w546, "koeff. cluster"="Coeff_cl_ch1") -> ("T solvation"=→"T1":dbl, "meas_voltage"=→"R1":dbl, "error out"=w547:errorcluster)  [unwired: 22 in]
          }
        }
        n210 = call "String_match (SubVI).vi"("channel id"="^b" ("regular expression"), "input string"=w422, "error in"=w388) -> ("match ?"=w402:i32, "output string"=w399:string, "match substring"=w400:string, "error out"=w401:errorcluster)  [unwired: 13 in]
        n211 = case shown="1, Default" w402 {
          tunnel: [w533 w539] -> w387
          tunnel: w401 -> [w533 w538]
          tunnel: w400 -> [_ w537]
          tunnel: w399 -> [w532 _]
          tunnel: [w532 _] -> w421
          frame -1 {
          }
          frame 1, Default {
            n212 = call "Volts_to_temperature_(SubVI).vi"("ch_data_string"=w537, "error in"=w538, "koeff. cluster"="Coeff_cl_ch2") -> ("T solvation"=→"T2":dbl, "meas_voltage"=→"R2":dbl, "error out"=w539:errorcluster)  [unwired: 22 in]
          }
        }
        n213 = call "String_match (SubVI).vi"("channel id"="^c" ("regular expression"), "input string"=w421, "error in"=w387) -> ("match ?"=w396:i32, "output string"=w395:string, "match substring"=w394:string, "error out"=w398:errorcluster)  [unwired: 13 in]
        n214 = case shown="1, Default" w396 {
          tunnel: w398 -> [w525 w531]
          tunnel: [w525 w530] -> w386
          tunnel: [w524 _] -> w420
          tunnel: w395 -> [w524 _]
          tunnel: w394 -> [_ w529]
          frame -1 {
          }
          frame 1, Default {
            n215 = call "Volts_to_temperature_(SubVI).vi"("ch_data_string"=w529, "error in"=w531, "koeff. cluster"="Coeff_cl_ch3") -> ("T solvation"=→"T3":dbl, "meas_voltage"=→"R3":dbl, "error out"=w530:errorcluster)  [unwired: 22 in]
          }
        }
        n216 = call "String_match (SubVI).vi"("channel id"="^d" ("regular expression"), "input string"=w420, "error in"=w386) -> ("match ?"=w391:i32, "output string"=w389:string, "match substring"=w390:string, "error out"=w392:errorcluster)  [unwired: 13 in]
        n217 = case shown="1, Default" w391 {
          tunnel: w392 -> [w517 w523]
          tunnel: [w517 w522] -> w385
          tunnel: w390 -> [_ w520]
          tunnel: w389 -> [w516 _]
          tunnel: [w516 _] -> w384
          frame -1 {
          }
          frame 1, Default {
            n218 = call "Volts_to_temperature_(SubVI).vi"("ch_data_string"=w520, "error in"=w523, "koeff. cluster"="Coeff_cl_ch4") -> ("T solvation"=→"T4":dbl, "meas_voltage"=→"R4":dbl, "error out"=w522:errorcluster)  [unwired: 22 in]
          }
        }
        n219 = call "String_match (SubVI).vi"("channel id"="^e" ("regular expression"), "input string"=w384, "error in"=w385) -> ("match ?"=w362:i32, "output string"=w365:string, "match substring"=w364:string, "error out"=w363:errorcluster)  [unwired: 13 in]
        n220 = case shown="1, Default" w362 {
          tunnel: [w509 w515] -> w381
          tunnel: w363 -> [w509 w514]
          tunnel: w364 -> [_ w513]
          tunnel: [w508 _] -> w358
          tunnel: w365 -> [w508 _]
          frame -1 {
          }
          frame 1, Default {
            n221 = call "Volts_to_temperature_(SubVI).vi"("ch_data_string"=w513, "error in"=w514, "koeff. cluster"="Coeff_cl_ch5") -> ("T solvation"=→"T5":dbl, "meas_voltage"=→"R5":dbl, "error out"=w515:errorcluster)  [unwired: 22 in]
          }
        }
        n222 = call "String_match (SubVI).vi"("channel id"="^f" ("regular expression"), "input string"=w358, "error in"=w381) -> ("match ?"=w367:i32, "output string"=w370:string, "match substring"=w369:string, "error out"=w368:errorcluster)  [unwired: 13 in]
        n223 = case shown="1, Default" w367 {
          tunnel: [w501 w507] -> w382
          tunnel: w368 -> [w501 w506]
          tunnel: w369 -> [_ w505]
          tunnel: w370 -> [w500 _]
          tunnel: [w500 _] -> w359
          frame -1 {
          }
          frame 1, Default {
            n224 = call "Volts_to_temperature_(SubVI).vi"("ch_data_string"=w505, "error in"=w506, "koeff. cluster"="Coeff_cl_ch6") -> ("T solvation"=→"T6":dbl, "meas_voltage"=→"R6":dbl, "error out"=w507:errorcluster)  [unwired: 22 in]
          }
        }
        n225 = call "String_match (SubVI).vi"("channel id"="^g" ("regular expression"), "input string"=w359, "error in"=w382) -> ("match ?"=w373:i32, "output string"=w374:string, "match substring"=w375:string, "error out"=w371:errorcluster)  [unwired: 13 in]
        n226 = case shown="1, Default" w373 {
          tunnel: w371 -> [w493 w499]
          tunnel: [w493 w498] -> w383
          tunnel: [w492 _] -> w360
          tunnel: w374 -> [w492 _]
          tunnel: w375 -> [_ w497]
          frame -1 {
          }
          frame 1, Default {
            n227 = call "Volts_to_temperature_(SubVI).vi"("ch_data_string"=w497, "error in"=w499, "koeff. cluster"="Coeff_cl_ch7") -> ("T solvation"=→"T7":dbl, "meas_voltage"=→"R7":dbl, "error out"=w498:errorcluster)  [unwired: 22 in]
          }
        }
        n228 = call "String_match (SubVI).vi"("channel id"="^h" ("regular expression"), "input string"=w360, "error in"=w383) -> ("match ?"=w378:i32, "output string"=w380:string, "match substring"=w379:string, "error out"=w377:errorcluster)  [unwired: 13 in]
        n229 = case shown="1, Default" w378 {
          tunnel: w377 -> [w423 w431]
          tunnel: w379 -> [_ w430]
          tunnel: w380 -> [_ _]
          tunnel: [w423 w424] -> w356
          frame -1 {
          }
          frame 1, Default {
            # "Все 8 каналов \nпрочитаны,\nвыводим показания \nна графики и \nсохраняем в файл"
            n230 = local read "File header exist?"() -> (w426:bool)
            n231 = call "Volts_to_temperature_(SubVI).vi"("ch_data_string"=w430, "error in"=w431, "koeff. cluster"="Coeff_cl_ch8") -> ("T solvation"=→"T8":dbl, "meas_voltage"=→"R8":dbl, "error out"=w425:errorcluster)  [unwired: 22 in]
            n232 = case shown="True" w426 {
              tunnel: [w436 w481] -> w424
              tunnel: w425 -> [_ w438]
              frame False {
                # "выполняется 1 раз"
                # "создание заголовка файла"
                n233 = call "Ch_data_title_pattern (SubVI).vi"("Единица измерений"="") -> ("error out"=w436:errorcluster, "Path"=→"Расположение файла":path, "Byte Stream File out"=→"refnum out":refnum<file>)  [unwired: 8 in]
                n234 = local write "File header exist?"(TRUE ("flag1")) -> ()
              }
              frame True {
                # "Сохранение результатов измерений и вывод на графики"
                n235 = local read "R2"() -> (w479:dbl)
                n236 = local read "R3"() -> (w478:dbl)
                n237 = local read "R4"() -> (w477:dbl)
                n238 = local read "R7"() -> (w474:dbl)
                n239 = local read "R1"() -> (w480:dbl)
                n240 = local read "R5"() -> (w476:dbl)
                n241 = local read "T1"() -> (w464:dbl)
                n242 = local read "T5"() -> (w460:dbl)
                n243 = local read "R6"() -> (w439:dbl)
                n244 = local read "R8"() -> (w475:dbl)
                n245 = local read "T2"() -> (w463:dbl)
                n246 = local read "T3"() -> (w462:dbl)
                n247 = local read "T4"() -> (w461:dbl)
                n248 = local read "T6"() -> (w459:dbl)
                n249 = local read "T7"() -> (w458:dbl)
                n250 = local read "T8"() -> (w457:dbl)
                n251 = Bundle("R1"=w480, "R2"=w479, "R3"=w478, "R4"=w477, "R5"=w476, "R6"=w439, "R7"=w474, "R8"=w475) -> (w465:T8)  [unwired: 1 in]
                n252 = Bundle("T1"=w464, "T2"=w463, "T3"=w462, "T4"=w461, "T5"=w460, "T6"=w459, "T7"=w458, "T8"=w457) -> (w437:T9)  [unwired: 1 in]
                n253 = Unbundle(w465) -> ("R1"=w473:dbl, "R2"=w472:dbl, "R3"=w471:dbl, "R4"=w470:dbl, "R5"=w469:dbl, "R6"=w468:dbl, "R7"=w467:dbl, "R8"=w466:dbl)
                n254 = Unbundle(w437) -> ("T1"=w449:dbl, "T2"=w450:dbl, "T3"=w451:dbl, "T4"=w452:dbl, "T5"=w453:dbl, "T6"=w454:dbl, "T7"=w455:dbl, "T8"=w456:dbl)
                n255 = local read "refnum out"() -> (w482:refnum<file>)
                n256 = call "Ch_data_pattern_8_save (SubVI).vi"("error in"=w438, "T Cluster"=w437, "R Cluster"=w465, "file"=w482) -> ("error out"=w481:errorcluster)  [unwired: 23 in]
                n257 = Merge Signals(w473) -> (w490:dynamicdata)
                n258 = Merge Signals(w472) -> (w489:dynamicdata)
                n259 = Merge Signals(w471) -> (w488:dynamicdata)
                n260 = Merge Signals(w470) -> (w491:dynamicdata)
                n261 = Merge Signals(w469) -> (w485:dynamicdata)
                n262 = Merge Signals(w468) -> (w484:dynamicdata)
                n263 = Merge Signals(w467) -> (w483:dynamicdata)
                n264 = Merge Signals(w466) -> (w486:dynamicdata)
                n265 = Merge Signals(w449) -> (w442:dynamicdata)
                n266 = Merge Signals(w450) -> (w443:dynamicdata)
                n267 = Merge Signals(w451) -> (w444:dynamicdata)
                n268 = Merge Signals(w452) -> (w441:dynamicdata)
                n269 = Merge Signals(w453) -> (w446:dynamicdata)
                n270 = Merge Signals(w454) -> (w447:dynamicdata)
                n271 = Merge Signals(w455) -> (w448:dynamicdata)
                n272 = Merge Signals(w456) -> (w445:dynamicdata)
                n273 = Merge Signals(w490, w489, w488, w491, w485, w484, w483, w486) -> (→"Graphs R":dynamicdata)
                n274 = Merge Signals(w442, w443, w444, w441, w446, w447, w448, w445) -> (→"Graphs T":dynamicdata)
              }
            }
          }
        }
      }
      frame True {
      }
    }
    n275 = local read "disconnected"() -> (w310:bool)
    n276 = case shown="False" w310 {
      tunnel: [w341 FALSE] -> w316
      tunnel: w309 -> [w340 _]
      frame False {
        n277 = Unbundle By Name(w340) -> ("status"=w342:bool)
        n278 = Not(x=w342) -> (.not. x?=w341:bool)
      }
      frame True {
      }
    }
    "Связь с прибором" <- w316
    n279 = property on="Graphs R" class="WFChart (strict)"("Active Plot"=w307) -> (error out=w332:errorcluster)  [unwired: 2 in, 1 out]
    n280 = property on="Graphs T" class="WFChart (strict)"("Active Plot"=w307) -> (error out=w308:errorcluster)  [unwired: 2 in, 1 out]
    n281 = property on="Graphs R" class="WFChart (strict)"(error in=w332, "Plot.Visible?"="1_ch_visible") -> (error out=w334:errorcluster)  [unwired: 1 in, 1 out]
    n282 = property on="Graphs T" class="WFChart (strict)"(error in=w308, "Plot.Visible?"="1_ch_visible") -> (error out=w301:errorcluster)  [unwired: 1 in, 1 out]
    n283 = property on="Graphs R" class="WFChart (strict)"(error in=w334, "Active Plot"=w302) -> (error out=w333:errorcluster)  [unwired: 1 in, 1 out]
    n284 = property on="Graphs T" class="WFChart (strict)"(error in=w301, "Active Plot"=w302) -> (error out=w305:errorcluster)  [unwired: 1 in, 1 out]
    n285 = property on="Graphs R" class="WFChart (strict)"(error in=w333, "Plot.Visible?"="2_ch_visible") -> (error out=w335:errorcluster)  [unwired: 1 in, 1 out]
    n286 = property on="Graphs T" class="WFChart (strict)"(error in=w305, "Plot.Visible?"="2_ch_visible") -> (error out=w298:errorcluster)  [unwired: 1 in, 1 out]
    n287 = property on="Graphs R" class="WFChart (strict)"(error in=w335, "Active Plot"=w299) -> (error out=w321:errorcluster)  [unwired: 1 in, 1 out]
    n288 = property on="Graphs T" class="WFChart (strict)"(error in=w298, "Active Plot"=w299) -> (error out=w304:errorcluster)  [unwired: 1 in, 1 out]
    n289 = property on="Graphs T" class="WFChart (strict)"(error in=w304, "Plot.Visible?"="3_ch_visible") -> (error out=w295:errorcluster)  [unwired: 1 in, 1 out]
    n290 = property on="Graphs R" class="WFChart (strict)"(error in=w321, "Plot.Visible?"="3_ch_visible") -> (error out=w322:errorcluster)  [unwired: 1 in, 1 out]
    n291 = property on="Graphs R" class="WFChart (strict)"(error in=w322, "Active Plot"=w296) -> (error out=w323:errorcluster)  [unwired: 1 in, 1 out]
    n292 = property on="Graphs T" class="WFChart (strict)"(error in=w295, "Active Plot"=w296) -> (error out=w303:errorcluster)  [unwired: 1 in, 1 out]
    n293 = property on="Graphs R" class="WFChart (strict)"(error in=w323, "Plot.Visible?"="4_ch_visible") -> (error out=w331:errorcluster)  [unwired: 1 in, 1 out]
    n294 = property on="Graphs T" class="WFChart (strict)"(error in=w303, "Plot.Visible?"="4_ch_visible") -> (error out=w285:errorcluster)  [unwired: 1 in, 1 out]
    n295 = property on="Graphs R" class="WFChart (strict)"(error in=w331, "Active Plot"=w286) -> (error out=w330:errorcluster)  [unwired: 1 in, 1 out]
    n296 = property on="Graphs T" class="WFChart (strict)"(error in=w285, "Active Plot"=w286) -> (error out=w287:errorcluster)  [unwired: 1 in, 1 out]
    n297 = property on="Graphs R" class="WFChart (strict)"(error in=w330, "Plot.Visible?"="5_ch_visible") -> (error out=w328:errorcluster)  [unwired: 1 in, 1 out]
    n298 = property on="Graphs T" class="WFChart (strict)"(error in=w287, "Plot.Visible?"="5_ch_visible") -> (error out=w291:errorcluster)  [unwired: 1 in, 1 out]
    n299 = property on="Graphs R" class="WFChart (strict)"(error in=w328, "Active Plot"=w283) -> (error out=w329:errorcluster)  [unwired: 1 in, 1 out]
    n300 = property on="Graphs T" class="WFChart (strict)"(error in=w291, "Active Plot"=w283) -> (error out=w288:errorcluster)  [unwired: 1 in, 1 out]
    n301 = property on="Graphs R" class="WFChart (strict)"(error in=w329, "Plot.Visible?"="6_ch_visible") -> (error out=w326:errorcluster)  [unwired: 1 in, 1 out]
    n302 = property on="Graphs T" class="WFChart (strict)"(error in=w288, "Plot.Visible?"="6_ch_visible") -> (error out=w292:errorcluster)  [unwired: 1 in, 1 out]
    n303 = property on="Graphs R" class="WFChart (strict)"(error in=w326, "Active Plot"=w281) -> (error out=w327:errorcluster)  [unwired: 1 in, 1 out]
    n304 = property on="Graphs T" class="WFChart (strict)"(error in=w292, "Active Plot"=w281) -> (error out=w289:errorcluster)  [unwired: 1 in, 1 out]
    n305 = property on="Graphs R" class="WFChart (strict)"(error in=w327, "Plot.Visible?"="7_ch_visible") -> (error out=w324:errorcluster)  [unwired: 1 in, 1 out]
    n306 = property on="Graphs T" class="WFChart (strict)"(error in=w289, "Plot.Visible?"="7_ch_visible") -> (error out=w293:errorcluster)  [unwired: 1 in, 1 out]
    n307 = property on="Graphs R" class="WFChart (strict)"(error in=w324, "Active Plot"=w279) -> (error out=w325:errorcluster)  [unwired: 1 in, 1 out]
    n308 = property on="Graphs T" class="WFChart (strict)"(error in=w293, "Active Plot"=w279) -> (error out=w290:errorcluster)  [unwired: 1 in, 1 out]
    n309 = property on="Graphs R" class="WFChart (strict)"(error in=w325, "Plot.Visible?"="8_ch_visible") -> ()  [unwired: 1 in, 2 out]
    n310 = property on="Graphs T" class="WFChart (strict)"(error in=w290, "Plot.Visible?"="8_ch_visible") -> ()  [unwired: 1 in, 2 out]
    n311 = local read "Связь с прибором"() -> (w313:bool)
    n312 = And(x="disconnect", y=w313) -> (x .and. y?=w314:bool)
    n313 = case shown="True" w314 {
      tunnel: w277 -> [w344 w348]
      tunnel: [w344 w347] -> w312
      frame False {
      }
      frame True {
        n314 = local read "connection ID"() -> (w345:refnum<k5>)
        n315 = TCP Close Connection(connection ID=w345, error in (no error)=w348) -> (error out=w347:errorcluster)  [unwired: 2 out]
        "disconnected" <- TRUE ("disconnected")
      }
    }
    n316 = call <vilib>:"General Error Handler.vi"("type of dialog (OK msg:1)"=u32 0 ("milliseconds to wait"), "error in (no error)"=w312) -> ()  [unwired: 14 out]
  }
  n317 = property on="сек." class="Str"("Disabled"=w30) -> (error out=w28:errorcluster)  [unwired: 2 in, 1 out]
  n318 = local write "Configuring ADC?"(FALSE ("TCP_Wr_fl")) -> ()
  n319 = property on="Coeff_cl_ch2" class="Clust (strict)"("Value"=w3) -> ()  [unwired: 2 in, 2 out]
  n320 = property on="Coeff_cl_ch1" class="Clust (strict)"("Value"=w3) -> ()  [unwired: 2 in, 2 out]
  n321 = property on="Coeff_cl_ch7" class="Clust (strict)"("Value"=w3) -> ()  [unwired: 2 in, 2 out]
  n322 = property on="Coeff_cl_ch5" class="Clust (strict)"("Value"=w3) -> ()  [unwired: 2 in, 2 out]
  n323 = property on="Coeff_cl_ch3" class="Clust (strict)"("Value"=w3) -> ()  [unwired: 2 in, 2 out]
  n324 = property on="Coeff_cl_ch8" class="Clust (strict)"("Value"=w3) -> ()  [unwired: 2 in, 2 out]
  n325 = property on="Coeff_cl_ch4" class="Clust (strict)"("Value"=w3) -> ()  [unwired: 2 in, 2 out]
  n326 = property on="Coeff_cl_ch6" class="Clust (strict)"("Value"=w3) -> ()  [unwired: 2 in, 2 out]
  n327 = property on="Расположение\n файла" class="Path"("Value"=path "" ("Расположение\n файла")) -> ()  [unwired: 2 in, 2 out]
  n328 = invoke on="Graphs R" class="WFChart (strict)" method="Reinit To Default"() -> (error out=w23:errorcluster)  [unwired: 3 in, 2 out]
  n329 = property on="мин." class="Str"(error in=w28, "Disabled"=w30) -> (error out=w27:errorcluster)  [unwired: 1 in, 1 out]
  n330 = Index Array(array=w15, index=1) -> (element=w16:refnum<vi>)
  n331 = property on="Graphs T" class="WFChart (strict)"("XScale.Minimum"=w6) -> (error out=w4:errorcluster)  [unwired: 2 in, 1 out]
  n332 = property class="Page"(reference=w16, "PageEnb"=T4."Page Disabled & Grayed" ("Page Enabled State")) -> ()  [unwired: 1 in, 2 out]
  n333 = property on="часы" class="Str"(error in=w27, "Disabled"=w30) -> (error out=w26:errorcluster)  [unwired: 1 in, 1 out]
  n334 = property on="Graphs R" class="WFChart (strict)"(error in=w23, "Value"=dynamicdata [{"t0"=timestamp(3465273261.7246556 s since 1904-01-01), "dt"=1.0, "Y"=[0.1931097262457384]}, {"t0"=timestamp(3465273261.7246556 s since 1904-01-01), "dt"=1.0, "Y"=[0.3594116459482981]}, {"t0"=timestamp(3465273261.7246556 s since 1904-01-01), "dt"=1.0, "Y"=[0.8898205452798131]}, {"t0"=timestamp(3465273261.7246556 s since 1904-01-01), "dt"=1.0, "Y"=[0.747699236883661]}] ("Graphs")) -> (error out=w25:errorcluster)  [unwired: 1 in, 1 out]
  n335 = property on="Graphs R" class="WFChart (strict)"(error in=w4) -> ("XScale.Maximum"=w5:dbl)  [unwired: 1 in, 2 out]
  n336 = invoke on="Добавить время" class="Ring (strict)" method="Reinit To Default"(error in=w26) -> (error out=w14:errorcluster)  [unwired: 2 in, 2 out]
  n337 = property on="Graphs R" class="WFChart (strict)"(error in=w25, "History Data"=dynamicdata[] []) -> (error out=w20:errorcluster)  [unwired: 1 in, 1 out]
  n338 = property on="Graphs R" class="WFChart (strict)"(error in=w20, "XScale.ScaleFit"=u8 0 ("Y Scale.Scale Fit")) -> (error out=w13:errorcluster)  [unwired: 1 in, 1 out]
  n339 = property on="Graphs T" class="WFChart (strict)"("XScale.Maximum"=w5) -> ()  [unwired: 2 in, 2 out]
  n340 = invoke on="File header exist?" class="Bool (strict)" method="Reinit To Default"(error in=w14) -> (error out=w24:errorcluster)  [unwired: 2 in, 2 out]
  n341 = invoke on="Graphs T" class="WFChart (strict)" method="Reinit To Default"(error in=w13) -> (error out=w9:errorcluster)  [unwired: 2 in, 2 out]
  n342 = property on="Расположение файла" class="Path"(error in=w24, "Disabled"=u8 2) -> ()  [unwired: 1 in, 2 out]
  n343 = property on="Graphs T" class="WFChart (strict)"(error in=w9, "Value"=dynamicdata [{"t0"=timestamp(3465273261.7246556 s since 1904-01-01), "dt"=1.0, "Y"=[0.1931097262457384]}, {"t0"=timestamp(3465273261.7246556 s since 1904-01-01), "dt"=1.0, "Y"=[0.3594116459482981]}, {"t0"=timestamp(3465273261.7246556 s since 1904-01-01), "dt"=1.0, "Y"=[0.8898205452798131]}, {"t0"=timestamp(3465273261.7246556 s since 1904-01-01), "dt"=1.0, "Y"=[0.747699236883661]}] ("Graphs")) -> (error out=w8:errorcluster)  [unwired: 1 in, 1 out]
  n344 = property on="Graphs R" class="WFChart (strict)"("YScale.ScaleFit"=w1) -> ()  [unwired: 2 in, 2 out]
  n345 = property on="Graphs T" class="WFChart (strict)"("YScale.ScaleFit"=w1) -> ()  [unwired: 2 in, 2 out]
  n346 = property on="Graphs T" class="WFChart (strict)"(error in=w8, "History Data"=dynamicdata[] []) -> (error out=w12:errorcluster)  [unwired: 1 in, 1 out]
  n347 = property on="Graphs T" class="WFChart (strict)"(error in=w12, "XScale.ScaleFit"=u8 0 ("Y Scale.Scale Fit")) -> ()  [unwired: 1 in, 2 out]
